vi "CB PWM Waveform Analysis.vi"(0 "Analysis Leg":i32, 1 "Board Selector":T1, 5 "Active Leg":i32, 7 "Duty Cycle":i32=25, 9 "Waveform":waveform(dbl)[](array[waveform])) -> (10 "Result (Boolean)":bool, 15 "Message":string)   [LabVIEW 2022 SP3]
uses:
  Serial Board Com/Board Select.ctl
  <vilib>/measure/mascope.llb/Pulse Measurements 1 chan.vi
  <vilib>/measure/madcrms.llb/Basic Averaged DC-RMS for 1 Chan.vi
  <vilib>/measure/NI_MAPro.lvlib
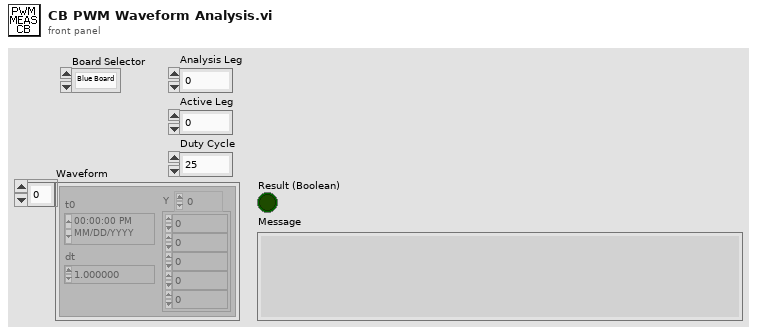
[diagram p1: front panel]
types:
  T1 = typedef "Board Select.ctl" = enum16{"Blue Board", "Green Board"}
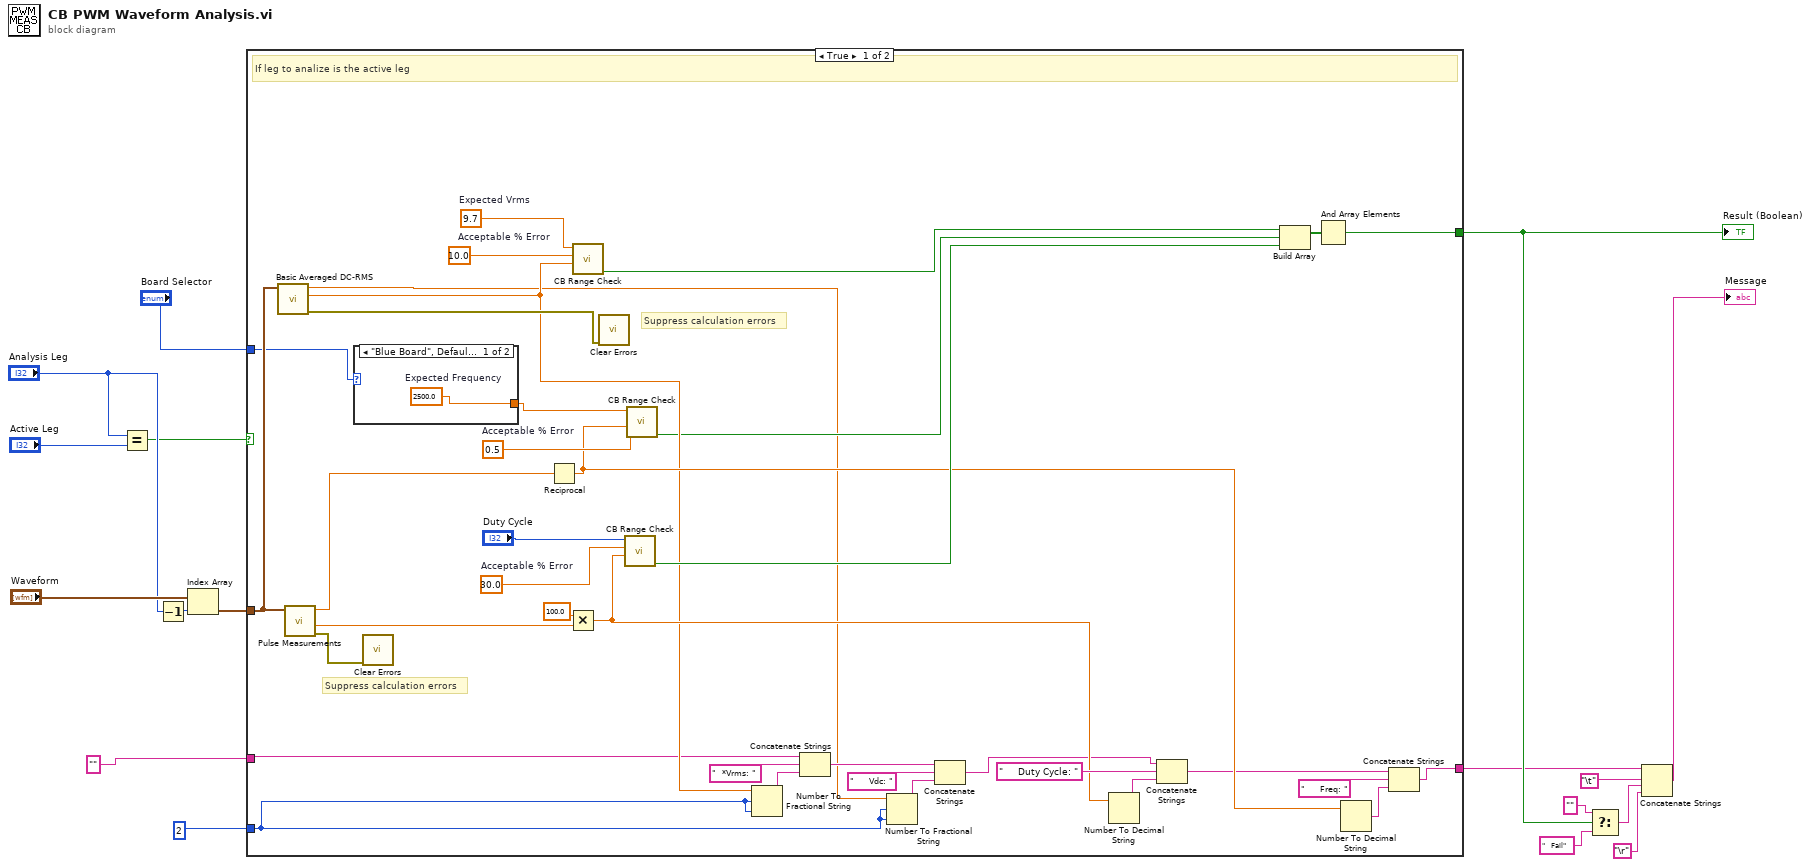
[diagram p0: block diagram]
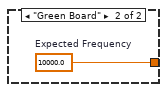
[diagram p2: hidden frame]
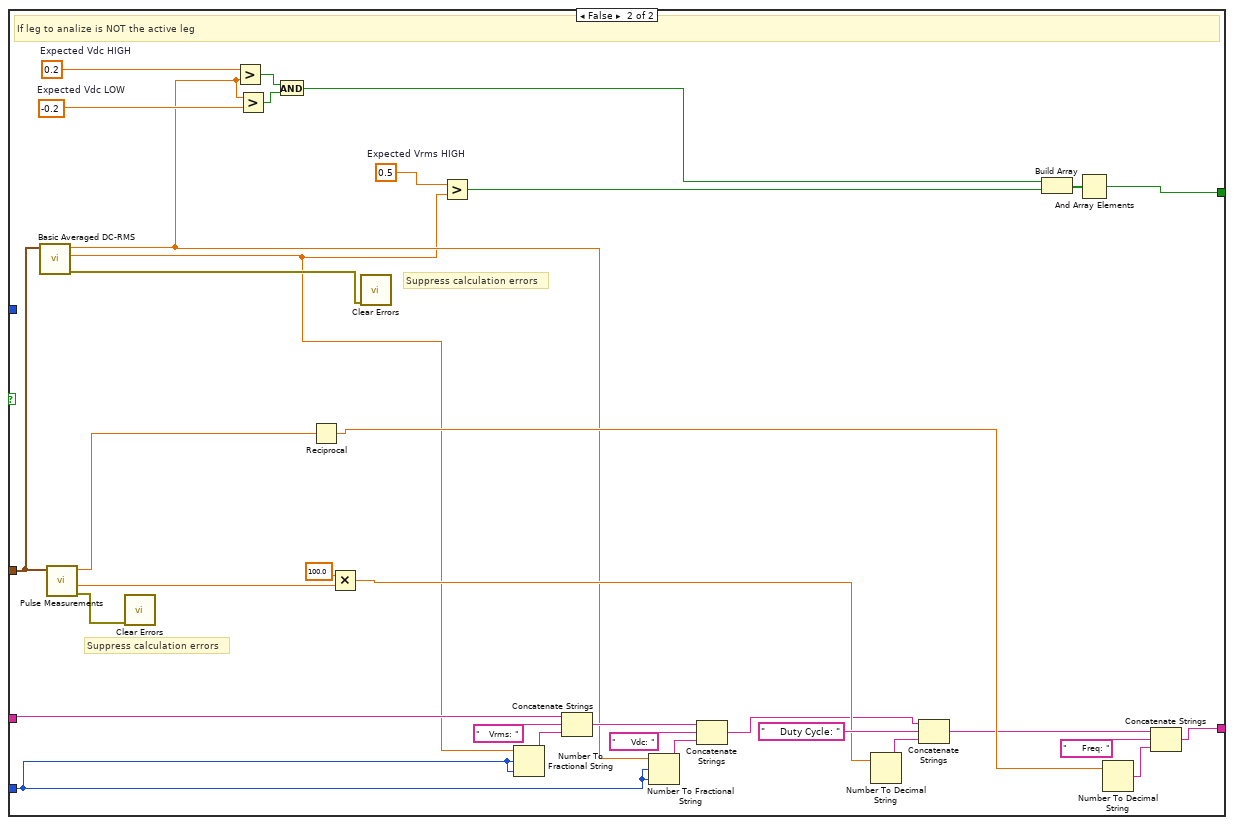
[diagram p3: hidden frame]
diagram:
  n1 = Equal?(x="Analysis Leg", y="Active Leg") -> (x = y?=w5:bool)
  n2 = Decrement(x="Analysis Leg") -> (x-1=w17:i32)
  n3 = Index Array(array="Waveform", index=w17) -> (element=w12:waveform(dbl))
  n4 = case shown="True" w5 {
    tunnel: w12 -> [w37 w76]
    tunnel: [w31 w73] -> w8
    tunnel: [w20 w60] -> w7
    tunnel: "" -> [w22 w62]
    tunnel: 2 -> [w19 w59]
    tunnel: "Board Selector" -> [w18 _]
    frame True {
      w25 = 10.0  # Acceptable % Error
      w24 = 9.7  # Expected Vrms
      w46 = 30.0  # Acceptable % Error
      w47 = 0.5  # Acceptable % Error
      # "Suppress calculation errors"
      # "Suppress calculation errors"
      # "If leg to analize is the active leg"
      n5 = call-poly <vilib>:"Basic Averaged DC-RMS.vi"("signal in"=w37) -> ("error out"=w38:errorcluster, "RMS value"=w33:dbl, "DC value"=w23:dbl)  [unwired: 7 in, 1 out]
      n6 = call-poly <vilib>:"Pulse Measurements.vi"("signal in"=w37) -> ("error out"=w48:errorcluster, "duty cycle"=w50:dbl, "period"=w49:dbl)  [unwired: 6 in, 2 out]
      n7 = case shown="\"Blue Board\", Default" w18 {
        tunnel: [w54 w55] -> w42
        frame "Blue Board", Default {
          w54 = 2500.0  # Expected Frequency
        }
        frame "Green Board" {
          w55 = 10000.0  # Expected Frequency
        }
      }
      n8 = call <vilib>:"Clear Errors.vi"("error in (no error)"=w48) -> ()  [unwired: 5 in, 2 out]
      n9 = Reciprocal(x=w49) -> (1/x=w39:dbl)
      n10 = Multiply(x=100.0, y=w50) -> (x*y=w43:dbl)
      n11 = call "CB Range Check.vi"("Actual Value"=w33, "Acceptable% Error"=w25, "Expected Value"=w24) -> ("Result (Boolean)"=w36:bool)  [unwired: 6 in, 2 out]
      n12 = call <vilib>:"Clear Errors.vi"("error in (no error)"=w38) -> ()  [unwired: 5 in, 2 out]
      n13 = call "CB Range Check.vi"("Actual Value"=w43, "Acceptable% Error"=w46, "Expected Value"="Duty Cycle") -> ("Result (Boolean)"=w51:bool)  [unwired: 6 in, 2 out]
      n14 = call "CB Range Check.vi"("Actual Value"=w39, "Acceptable% Error"=w47, "Expected Value"=w42) -> ("Result (Boolean)"=w32:bool)  [unwired: 6 in, 2 out]
      n15 = Number To Fractional String(number=w33, width (-)=w19, precision (6)=w19) -> (F-format string=w35:string)  [unwired: 1 in]
      n16 = Concatenate Strings(w22, "  *Vrms: " ("string"), w35) -> (w27:string)
      n17 = Number To Fractional String(number=w23, width (-)=w19, precision (6)=w19) -> (F-format string=w29:string)  [unwired: 1 in]
      n18 = Concatenate Strings(w27, "     Vdc: " ("string"), w29) -> (w21:string)
      n19 = Number To Decimal String(number=w43) -> (decimal integer string=w44:string)  [unwired: 1 in]
      n20 = Concatenate Strings(w21, "     Duty Cycle: " ("string"), w44) -> (w28:string)
      n21 = Build Array(w36, w32, w51) -> (w52:bool[])
      n22 = And Array Elements(Boolean array=w52) -> (logical AND=w31:bool)
      n23 = Number To Decimal String(number=w39) -> (decimal integer string=w40:string)  [unwired: 1 in]
      n24 = Concatenate Strings(w28, "     Freq: " ("string"), w40) -> (w20:string)
    }
    frame False {
      w58 = 0.5  # Expected Vrms HIGH
      w67 = -0.2  # Expected Vdc LOW
      w68 = 0.2  # Expected Vdc HIGH
      # "Suppress calculation errors"
      # "Suppress calculation errors"
      # "If leg to analize is NOT the active leg"
      n25 = call-poly <vilib>:"Basic Averaged DC-RMS.vi"("signal in"=w76) -> ("error out"=w77:errorcluster, "RMS value"=w57:dbl, "DC value"=w63:dbl)  [unwired: 7 in, 1 out]
      n26 = call-poly <vilib>:"Pulse Measurements.vi"("signal in"=w76) -> ("error out"=w84:errorcluster, "duty cycle"=w86:dbl, "period"=w85:dbl)  [unwired: 6 in, 2 out]
      n27 = call <vilib>:"Clear Errors.vi"("error in (no error)"=w84) -> ()  [unwired: 5 in, 2 out]
      n28 = Greater?(x=w68, y=w63) -> (0:w66:bool)
      n29 = Greater?(x=w63, y=w67) -> (0:w65:bool)
      n30 = And(x=w66, y=w65) -> (x .and. y?=w64:bool)
      n31 = Reciprocal(x=w85) -> (1/x=w78:dbl)
      n32 = Multiply(x=100.0, y=w86) -> (x*y=w81:dbl)
      n33 = call <vilib>:"Clear Errors.vi"("error in (no error)"=w77) -> ()  [unwired: 5 in, 2 out]
      n34 = Greater?(x=w58, y=w57) -> (0:w56:bool)
      n35 = Number To Fractional String(number=w57, width (-)=w59, precision (6)=w59) -> (F-format string=w75:string)  [unwired: 1 in]
      n36 = Concatenate Strings(w62, "   Vrms: " ("string"), w75) -> (w69:string)
      n37 = Number To Fractional String(number=w63, width (-)=w59, precision (6)=w59) -> (F-format string=w71:string)  [unwired: 1 in]
      n38 = Concatenate Strings(w69, "     Vdc: " ("string"), w71) -> (w61:string)
      n39 = Number To Decimal String(number=w81) -> (decimal integer string=w82:string)  [unwired: 1 in]
      n40 = Concatenate Strings(w61, "     Duty Cycle: " ("string"), w82) -> (w70:string)
      n41 = Build Array(w64, w56) -> (w87:bool[])
      n42 = And Array Elements(Boolean array=w87) -> (logical AND=w73:bool)
      n43 = Number To Decimal String(number=w78) -> (decimal integer string=w79:string)  [unwired: 1 in]
      n44 = Concatenate Strings(w70, "     Freq: " ("string"), w79) -> (w60:string)
    }
  }
  "Result (Boolean)" <- w8
  n45 = Select(t="" ("string"), s=w8, f="   Fail" ("string")) -> (s? t:f=w9:string)
  n46 = Concatenate Strings(w7, "\t", w9, "\r") -> (→"Message":string)
